vi "Streaming Example.vi"() -> ()   [LabVIEW 2020]
uses:
  g_industrial_cam/Device Enumeration.ctl
  g_industrial_cam/Camera/Camera.lvclass/Camera.ctl
  g_industrial_cam/Buffer/Buffer.lvclass/Buffer.ctl
  g_industrial_cam/Camera/GetSetTrigger.vi
  g_industrial_cam/Camera/GetSetPixelFormat.vi
  g_industrial_cam/Buffer/Access Handle.vi
  g_industrial_cam/Camera/Check Not Disconnected.vi
  <vilib>/Utility/error.llb/Error Cluster From Error Code.vi
  g_industrial_cam/Camera/Destroy Stream Events.vi
  g_industrial_cam/Camera/Check Stream OK.vi
  <vilib>/picture/picture.llb/Draw 8-Bit Pixmap.vi
  g_industrial_cam/Buffer/Buffer.lvclass
  g_industrial_cam/Camera/Camera.lvclass
panel:
  in  "stop 2":bool
  out "Frame-Error Count":u64
  out "Frame Count (inc Errors)":u64
  out "Pixel Format":string caption="Pixel Format (Only Mono 8 Decoding Supported in This Example)"
  out "Trigger Source":string
  out "Timeout":bool
  out "Devices":T1[](array[typedef])
  in  "Picture Zoom Factor":sgl
  out "Picture":picture
  in  "stop":bool
  out "error out":errorcluster
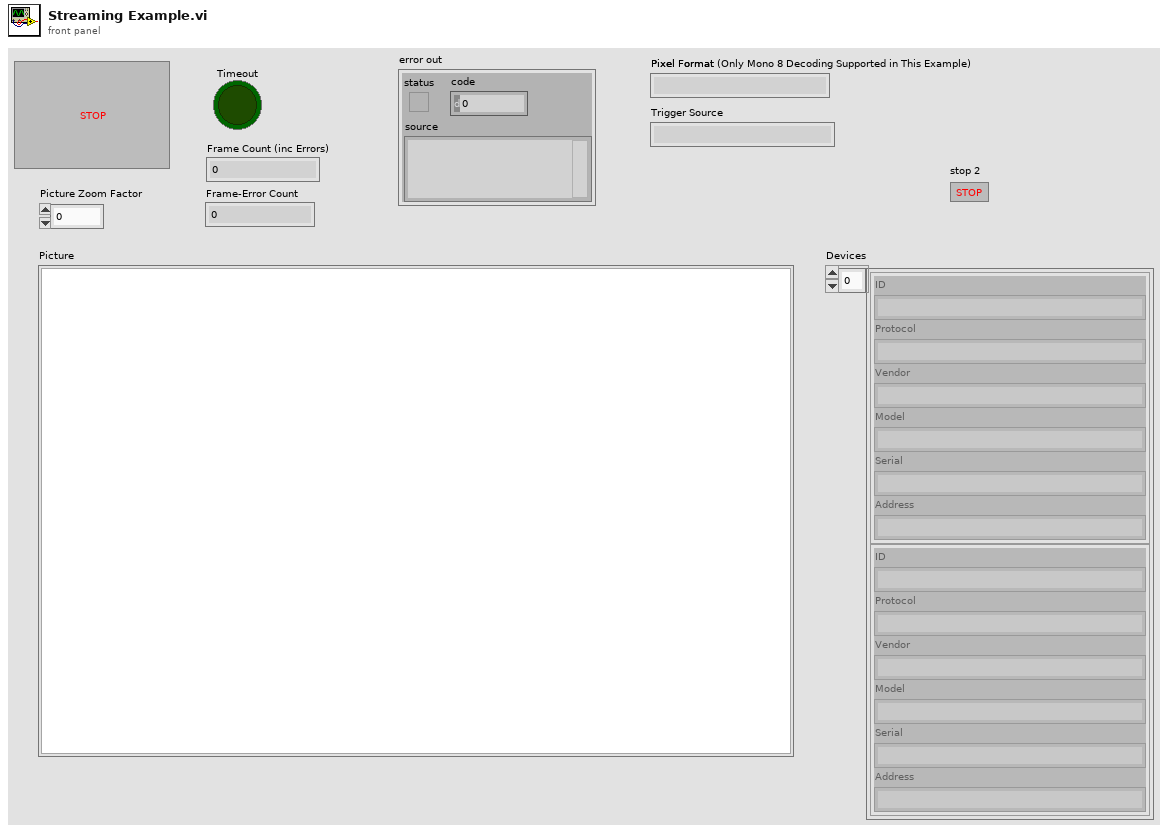
[diagram p1: front panel]
types:
  T1 = typedef "Device Enumeration.ctl" = cluster{"ID":string, "Protocol":string, "Vendor":string, "Model":string, "Serial":string, "Address":string}
  T2 = typedef "Buffer.lvclass/Image Size.ctl" = cluster{"Width":u16, "Height":u16}
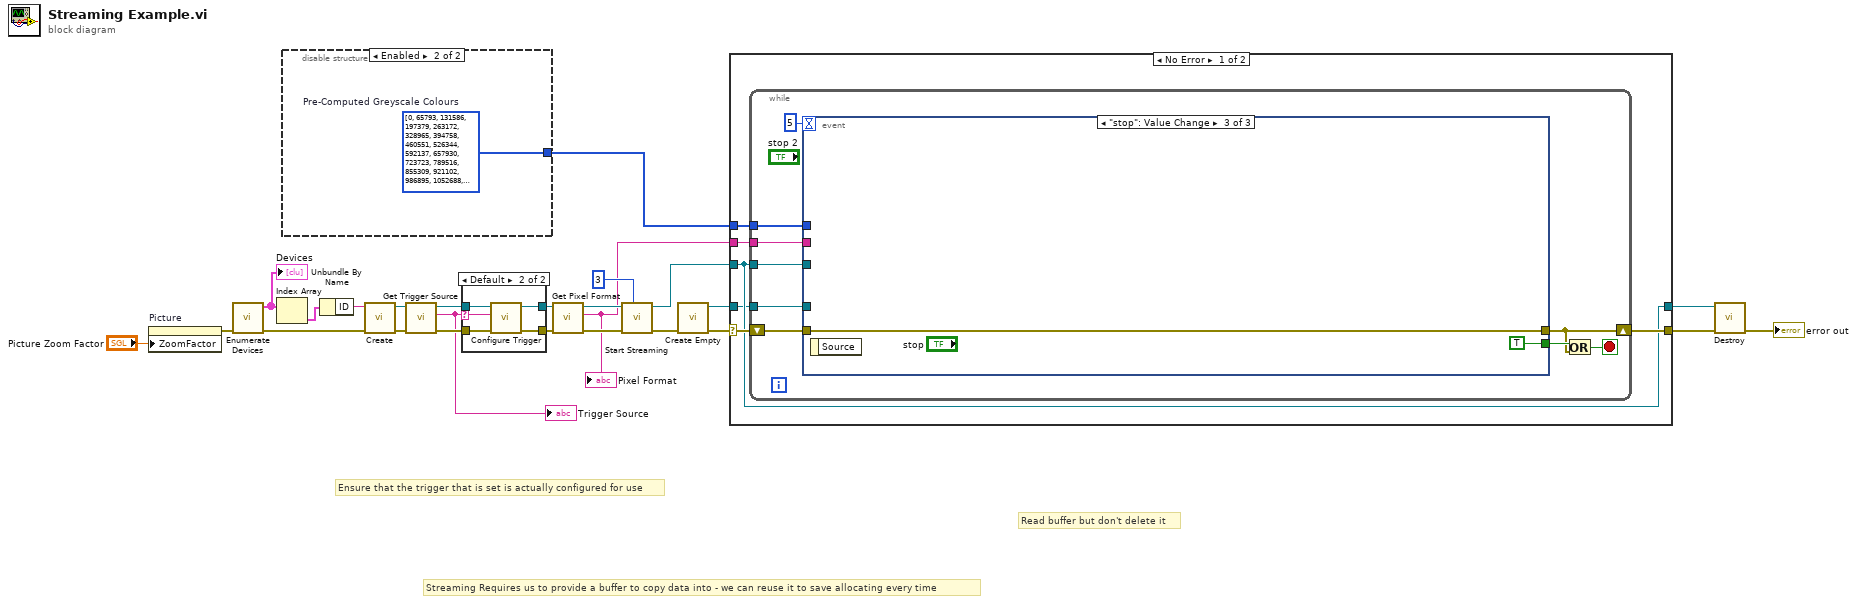
[diagram p0: block diagram]
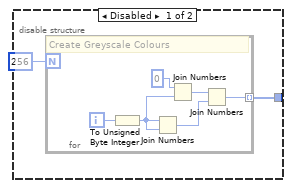
[diagram p3: hidden frame]
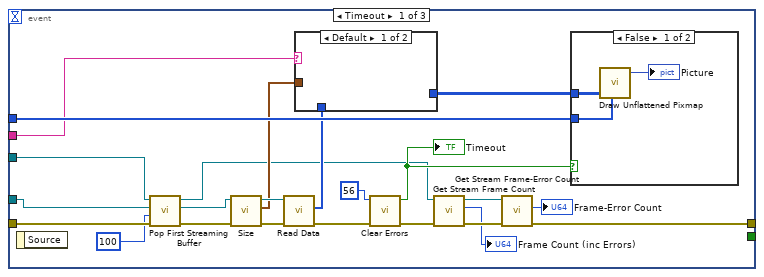
[diagram p4: hidden frame]
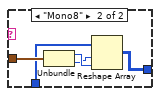
[diagram p5: hidden frame]
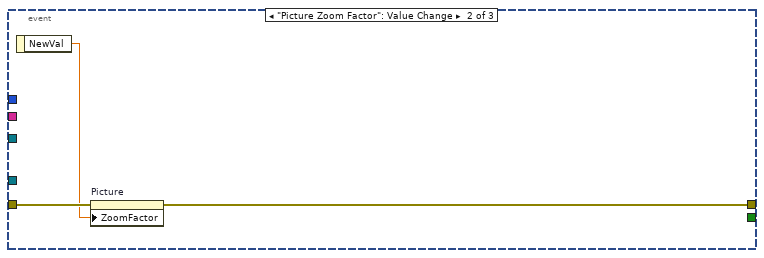
[diagram p7: hidden frame]
diagram:
  # "Ensure that the trigger that is set is actually configured for use"
  # "Read buffer but don't delete it"
  # "Streaming Requires us to provide a buffer to copy data into - we can reuse it to save allocating every time"
  n1 = property on="Picture" class="Pict"("ZoomFactor"="Picture Zoom Factor") -> (error out=w20:errorcluster)  [unwired: 2 in, 1 out]
  n2 = call "Enumerate Devices.vi"("error in (no error)"=w20) -> ("error out"=w23:errorcluster, "Devices"=w25:T1[])  [unwired: 9 in]
  "Devices" <- w25
  n3 = Index Array(array=w25) -> (element=w24:T1)  [unwired: 1 in]
  n4 = disable-structure shown="Enabled" {
    disable-tunnel: [w26 w34] -> w12
    frame Disabled {
      n5 = for {
        N: 256 -> [_]
        tunnel: [w28] -> w26 mode=indexing
        i -> [w33]
        # "Create Greyscale Colours"
        n6 = To Unsigned Byte Integer(number=w33) -> (unsigned 8bit integer=w32:u8)
        n7 = Join Numbers(hi=w32, lo=w32) -> ((hi.lo)=w29:u16)
        n8 = Join Numbers(hi=u8 0, lo=w32) -> ((hi.lo)=w30:u16)
        n9 = Join Numbers(hi=w30, lo=w29) -> ((hi.lo)=w28:u32)
      }
    }
    frame Enabled {
      w34 = u32[] [0, 65793, 131586, 197379, 263172, 328965, 394758, 460551, 526344, 592137, 657930, 723723, 789516, 855309, 921102, 986895, 1052688, 1118481, 1184274, 1250067, 1315860, 1381653, 1447446, 1513239, 1579032, 1644825, 1710618, 1776411, 1842204, 1907997, 1973790, 2039583, 2105376, 2171169, 2236962, 2302755, 2368548, 2434341, 2500134, 2565927, 2631720, 2697513, 2763306, 2829099, 2894892, 2960685, 3026478, 3092271, 3158064, 3223857, 3289650, 3355443, 3421236, 3487029, 3552822, 3618615, 3684408, 3750201, 3815994, 3881787, 3947580, 4013373, 4079166, 4144959, 4210752, 4276545, 4342338, 4408131, 4473924, 4539717, 4605510, 4671303, 4737096, 4802889, 4868682, 4934475, 5000268, 5066061, 5131854, 5197647, 5263440, 5329233, 5395026, 5460819, 5526612, 5592405, 5658198, 5723991, 5789784, 5855577, 5921370, 5987163, 6052956, 6118749, 6184542, 6250335, 6316128, 6381921, 6447714, 6513507, 6579300, 6645093, 6710886, 6776679, 6842472, 6908265, 6974058, 7039851, 7105644, 7171437, 7237230, 7303023, 7368816, 7434609, 7500402, 7566195, 7631988, 7697781, 7763574, 7829367, 7895160, 7960953, 8026746, 8092539, 8158332, 8224125, 8289918, 8355711, 8421504, 8487297, 8553090, 8618883, 8684676, 8750469, 8816262, 8882055, 8947848, 9013641, 9079434, 9145227, 9211020, 9276813, 9342606, 9408399, 9474192, 9539985, 9605778, 9671571, 9737364, 9803157, 9868950, 9934743, 10000536, 10066329, 10132122, 10197915, 10263708, 10329501, 10395294, 10461087, 10526880, 10592673, 10658466, 10724259, 10790052, 10855845, 10921638, 10987431, 11053224, 11119017, 11184810, 11250603, 11316396, 11382189, 11447982, 11513775, 11579568, 11645361, 11711154, 11776947, 11842740, 11908533, 11974326, 12040119, 12105912, 12171705, 12237498, 12303291, 12369084, 12434877, 12500670, 12566463, 12632256, 12698049, 12763842, 12829635, 12895428, 12961221, 13027014, 13092807, 13158600, 13224393, 13290186, 13355979, 13421772, 13487565, 13553358, 13619151, 13684944, 13750737, 13816530, 13882323, 13948116, 14013909, 14079702, 14145495, 14211288, 14277081, 14342874, 14408667, 14474460, 14540253, 14606046, 14671839, 14737632, 14803425, 14869218, 14935011, 15000804, 15066597, 15132390, 15198183, 15263976, 15329769, 15395562, 15461355, 15527148, 15592941, 15658734, 15724527, 15790320, 15856113, 15921906, 15987699, 16053492, 16119285, 16185078, 16250871, 16316664, 16382457, 16448250, 16514043, 16579836, 16645629, 16711422, 16777215]  # Pre-Computed Greyscale Colours
    }
  }
  n10 = Unbundle By Name(w24) -> ("ID"=w22:string)
  n11 = call "Create.vi"("error in (no error)"=w23, "Identifier (ID, IP etc)"=w22) -> ("error out"=w21:errorcluster, "Camera"=w14:refnum<class "Camera.lvclass">)  [unwired: 8 in]
  n12 = call "Get Trigger Source.vi"("error in (no error)"=w21, "Camera in"=w14) -> ("error out"=w13:errorcluster, "Trigger Source"=w2:string, "Camera"=w4:refnum<class "Camera.lvclass">)  [unwired: 7 in]
  "Trigger Source" <- w2
  n13 = case shown="Default" w2 {
    selector: w2 -> [_ w37]
    tunnel: w13 -> [w35 w41]
    tunnel: [w35 w40] -> w5
    tunnel: w4 -> [w36 w39]
    tunnel: [w36 w38] -> w3
    frame "" {
    }
    frame Default {
      n14 = call "Configure Trigger.vi"("error in (no error)"=w41, "Source"=w37, "Camera in"=w39) -> ("error out"=w40:errorcluster, "Camera"=w38:refnum<class "Camera.lvclass">)  [unwired: 7 in]
    }
  }
  n15 = call "Get Pixel Format.vi"("error in (no error)"=w5, "Camera in"=w3) -> ("error out"=w8:errorcluster, "Pixel Format"=w6:string, "Camera"=w7:refnum<class "Camera.lvclass">)  [unwired: 7 in]
  "Pixel Format" <- w6
  n16 = call "Start Streaming.vi"("Additional Buffers (Default: 3)"=u16 3 ("Additional Buffers (3)"), "error in (no error)"=w8, "Camera in"=w7) -> ("error out"=w18:errorcluster, "Camera"=w1:refnum<class "Camera.lvclass">)  [unwired: 7 in]
  n17 = call "Create Empty.vi"("error in (no error)"=w18) -> ("error out"=w17:errorcluster, "Buffer out"=w16:refnum<class "Buffer.lvclass">)  [unwired: 9 in]
  n18 = case shown="No Error" w17 {
    selector: w17 -> [w47 w93]
    tunnel: w1 -> [w45 w94]
    tunnel: [w46 w93] -> w10
    tunnel: [w45 w94] -> w11
    tunnel: w12 -> [w44 _]
    tunnel: w16 -> [w43 _]
    tunnel: w6 -> [w42 _]
    frame No Error {
      n19 = while {
        shift-right: [w51] -> w46
        shift-left: w47 -> [w50]
        tunnel: w45 -> [w56]
        tunnel: w44 -> [w53]
        tunnel: w43 -> [w52]
        tunnel: w42 -> [w48]
        stop <- w54 stop-if-true
        n20 = event shown="[2] \"stop\": Value Change" {
          selector: _ -> [_ _ _]
          dyn-events: _ -> [_ _ _]
          timeout: 5 -> [_ _ _]
          tunnel: w56 -> [w79 _ _]
          tunnel: w50 -> [w78 w90 w92]
          tunnel: [w62 w89 w92] -> w51
          tunnel: [_ _ TRUE] -> w55
          tunnel: w53 -> [w76 _ _]
          tunnel: w52 -> [w75 _ _]
          tunnel: w48 -> [w66 _ _]
          event Timeout {
            n21 = event-data() -> ()  [unwired: 1 in, 1 out]
            n22 = call "Pop First Streaming Buffer.vi"("error in (no error)"=w78, "Timeout (ms) Default: 10000"=100 ("Timeout (ms) Default: -1"), "Buffer in"=w75, "Camera in"=w79) -> ("error out"=w73:errorcluster, "Buffer"=w74:refnum<class "Buffer.lvclass">, "Camera"=w60:refnum<class "Camera.lvclass">)  [unwired: 5 in]
            n23 = call "Size.vi"("error in (no error)"=w73, "Buffer Data in"=w74) -> ("error out"=w72:errorcluster, "Image Size"=w65:T2, "Buffer Data"=w71:refnum<class "Buffer.lvclass">)  [unwired: 7 in]
            n24 = call "Read Data.vi"("error in (no error)"=w72, "Buffer in"=w71) -> ("error out"=w70:errorcluster, "Data"=w64:u8[])  [unwired: 7 in, 1 out]
            n25 = case shown="Default" w66 {
              tunnel: w65 -> [_ w84]
              tunnel: w64 -> [_ w81]
              tunnel: [_ w80] -> w63
              frame Default {
              }
              frame "Mono8" {
                n26 = Unbundle(w84) -> ("Width"=w83:u16, "Height"=w82:u16)
                n27 = Reshape Array(w81, w82, w83) -> (w80:u8[][])
              }
            }
            n28 = call <vilib>:"Clear Errors.vi"("error in (no error)"=w70, "specific error code to clear (0: all)"=56) -> ("error out"=w77:errorcluster, "specific error cleared?"=w67:bool)  [unwired: 4 in]
            "Timeout" <- w67
            n29 = call "Get Stream Frame Count.vi"("error in (no error)"=w77, "Camera in"=w60) -> ("error out"=w61:errorcluster, "Frame Count (inc Errors)"=→"Frame Count (inc Errors)":u64, "Camera"=w59:refnum<class "Camera.lvclass">)  [unwired: 7 in]
            n30 = call "Get Stream Frame-Error Count.vi"("error in (no error)"=w61, "Camera in"=w59) -> ("error out"=w62:errorcluster, "Frame-Error Count"=→"Frame-Error Count":u64)  [unwired: 7 in, 1 out]
            n31 = case shown="False" w67 {
              tunnel: w76 -> [w86 _]
              tunnel: w63 -> [w85 _]
              frame False {
                n32 = call-poly <vilib>:"Draw Unflattened Pixmap.vi"("data"=w85, "color table"=w86) -> ("new picture"=→"Picture":picture)  [unwired: 7 in]
              }
              frame True {
              }
            }
          }
          event "Picture Zoom Factor": Value Change {
            n33 = event-data() -> ("NewVal"=w88:sgl)  [unwired: 1 in]
            n34 = property on="Picture" class="Pict"(error in=w90, "ZoomFactor"=w88) -> (error out=w89:errorcluster)  [unwired: 1 in, 1 out]
          }
          event "stop": Value Change {
            n35 = event-data() -> ()  [unwired: 1 in, 1 out]
          }
        }
        n36 = Or(x=w55, y=w51) -> (x .or. y?=w54:bool)
      }
    }
    frame Error {
    }
  }
  n37 = call "Destroy.vi"("error in (no error)"=w10, "Camera in"=w11) -> ("error out"=→"error out":errorcluster)  [unwired: 9 in]
